vi "fp display engine.vi"(7 "channel data in":sgl[][][](array[numeric]), 10 "Image Refs In":T1[](array[typedef]), 11 "DisplayRefsIn(generic class)":refnum<vi>[](array[refnum])) -> ()   [LabVIEW 2017]
doc: "SciScan 1.2 160622"
uses:
  <vilib>/vision/Image Controls.llb/IMAQ Image.ctl
  Custom Controls/MAIN Image panel tab Control type def.ctl
  Custom Controls/Image Types.ctl
  Custom Controls/scan mode main settings tab.ctl
  Custom Controls/Ch selector.ctl
  GFG/GFGbooleanGet.vi
  GFG/GFGfpRefGet.vi
  <vilib>/vision/NI_Vision_Development_Module.lvlib
  GFG/GFG library.lvlib
panel:
  in  "ROI colors":u32[](array[colorbox])=[6618880, 16716362, 16860, 16776793, 16750848, 16448250, 16716530, 9567230, 16764108, 7340212, 32639, 0, 13816530, 8421376, 8421631, 7171459, 6618880, 16716362, 16860, 16776793, 16750848, 16448250, 16716530, 9567230, 16764108, 7340212, 32639, 0, 13816530, 8421376, 8421631, 7171459, 6618880, 16716362, 16860, 16776793, 16750848, 16448250, 16716530, 9567230, 16764108, 7340212, 32639, 0, 13816530, 8421376, 8421631, 7171459, 6618880, 16716362, 16860, 16776793, 16750848, 16448250, 16716530, 9567230, 16764108, 7340212, 32639, 0, 13816530, 8421376, 8421631, 7171459, 6618880, 16716362, 16860, 16776793, 16750848, 16448250, 16716530, 9567230, 16764108, 7340212, 32639, 0, 13816530, 8421376, 8421631, 7171459, 6618880, 16716362, 16860, 16776793, 16750848, 16448250, 16716530, 9567230, 16764108, 7340212, 32639, 0, 13816530, 8421376, 8421631, 7171459, 6618880, 16716362, 16860, 16776793, 16750848, 16448250, 16716530, 9567230, 16764108, 7340212, 32639, 0, 13816530, 8421376, 8421631, 7171459, 6618880, 16716362, 16860, 16776793, 16750848, 16448250, 16716530, 9567230, 16764108, 7340212, 32639, 0, 13816530, 8421376, 8421631, 7171459, 6618880, 16716362, 16860, 16776793, 16750848, 16448250, 16716530, 9567230, 16764108, 7340212, 32639, 0, 13816530, 8421376, 8421631, 7171459, 6618880, 16716362, 16860, 16776793, 16750848, 16448250, 16716530, 9567230, 16764108, 7340212, 32639, 0, 13816530, 8421376, 8421631, 7171459, 6618880, 16716362, 16860, 16776793, 16750848, 16448250, 16716530, 9567230, 16764108, 7340212, 32639, 0, 13816530, 8421376, 8421631, 7171459, 6618880, 16716362, 16860, 16776793, 16750848, 16448250, 16716530, 9567230, 16764108, 7340212, 32639, 0, 13816530, 8421376, 8421631, 7171459, 6618880, 16716362, 16860, 16776793, 16750848, 16448250, 16716530, 9567230, 16764108, 7340212, 32639, 0, 13816530, 8421376, 8421631, 7171459, 6618880, 16716362, 16860, 16776793, 16750848, 16448250, 16716530, 9567230, 16764108, 7340212, 32639, 0, 13816530, 8421376, 8421631, 7171459, 6618880, 16716362, 16860, 16776793, 16750848, 16448250, 16716530, 9567230, 16764108, 7340212, 32639, 0, 13816530, 8421376, 8421631, 7171459, 6618880, 16716362, 16860, 16776793, 16750848, 16448250, 16716530, 9567230, 16764108, 7340212, 32639, 0, 13816530, 8421376, 8421631, 7171459, 6618880, 16716362, 16860, 16776793, 16750848, 16448250, 16716530, 9567230, 16764108, 7340212, 32639, 0, 13816530, 8421376, 8421631, 7171459, 6618880, 16716362, 16860, 16776793, 16750848, 16448250, 16716530, 9567230, 16764108, 7340212, 32639, 0, 13816530, 8421376, 8421631, 7171459, 6618880, 16716362, 16860, 16776793, 16750848, 16448250, 16716530, 9567230, 16764108, 7340212, 32639, 0, 13816530, 8421376, 8421631, 7171459, 6618880, 16716362, 16860, 16776793, 16750848, 16448250, 16716530, 9567230, 16764108, 7340212, 32639, 0, 13816530, 8421376, 8421631, 7171459, 6618880, 16716362, 16860, 16776793, 16750848, 16448250, 16716530, 9567230, 16764108, 7340212, 32639, 0, 13816530, 8421376, 8421631, 7171459, 6618880, 16716362, 16860, 16776793, 16750848, 16448250, 16716530, 9567230, 16764108, 7340212, 32639, 0, 13816530, 8421376, 8421631, 7171459, 6618880, 16716362, 16860, 16776793, 16750848, 16448250, 16716530, 9567230, 16764108, 7340212, 32639, 0, 13816530, 8421376, 8421631, 7171459, 6618880, 16716362, 16860, 16776793, 16750848, 16448250, 16716530, 9567230, 16764108, 7340212, 32639, 0, 13816530, 8421376, 8421631, 7171459, 6618880, 16716362, 16860, 16776793, 16750848, 16448250, 16716530, 9567230, 16764108, 7340212, 32639, 0, 13816530, 8421376, 8421631, 7171459]
  out "error out":errorcluster
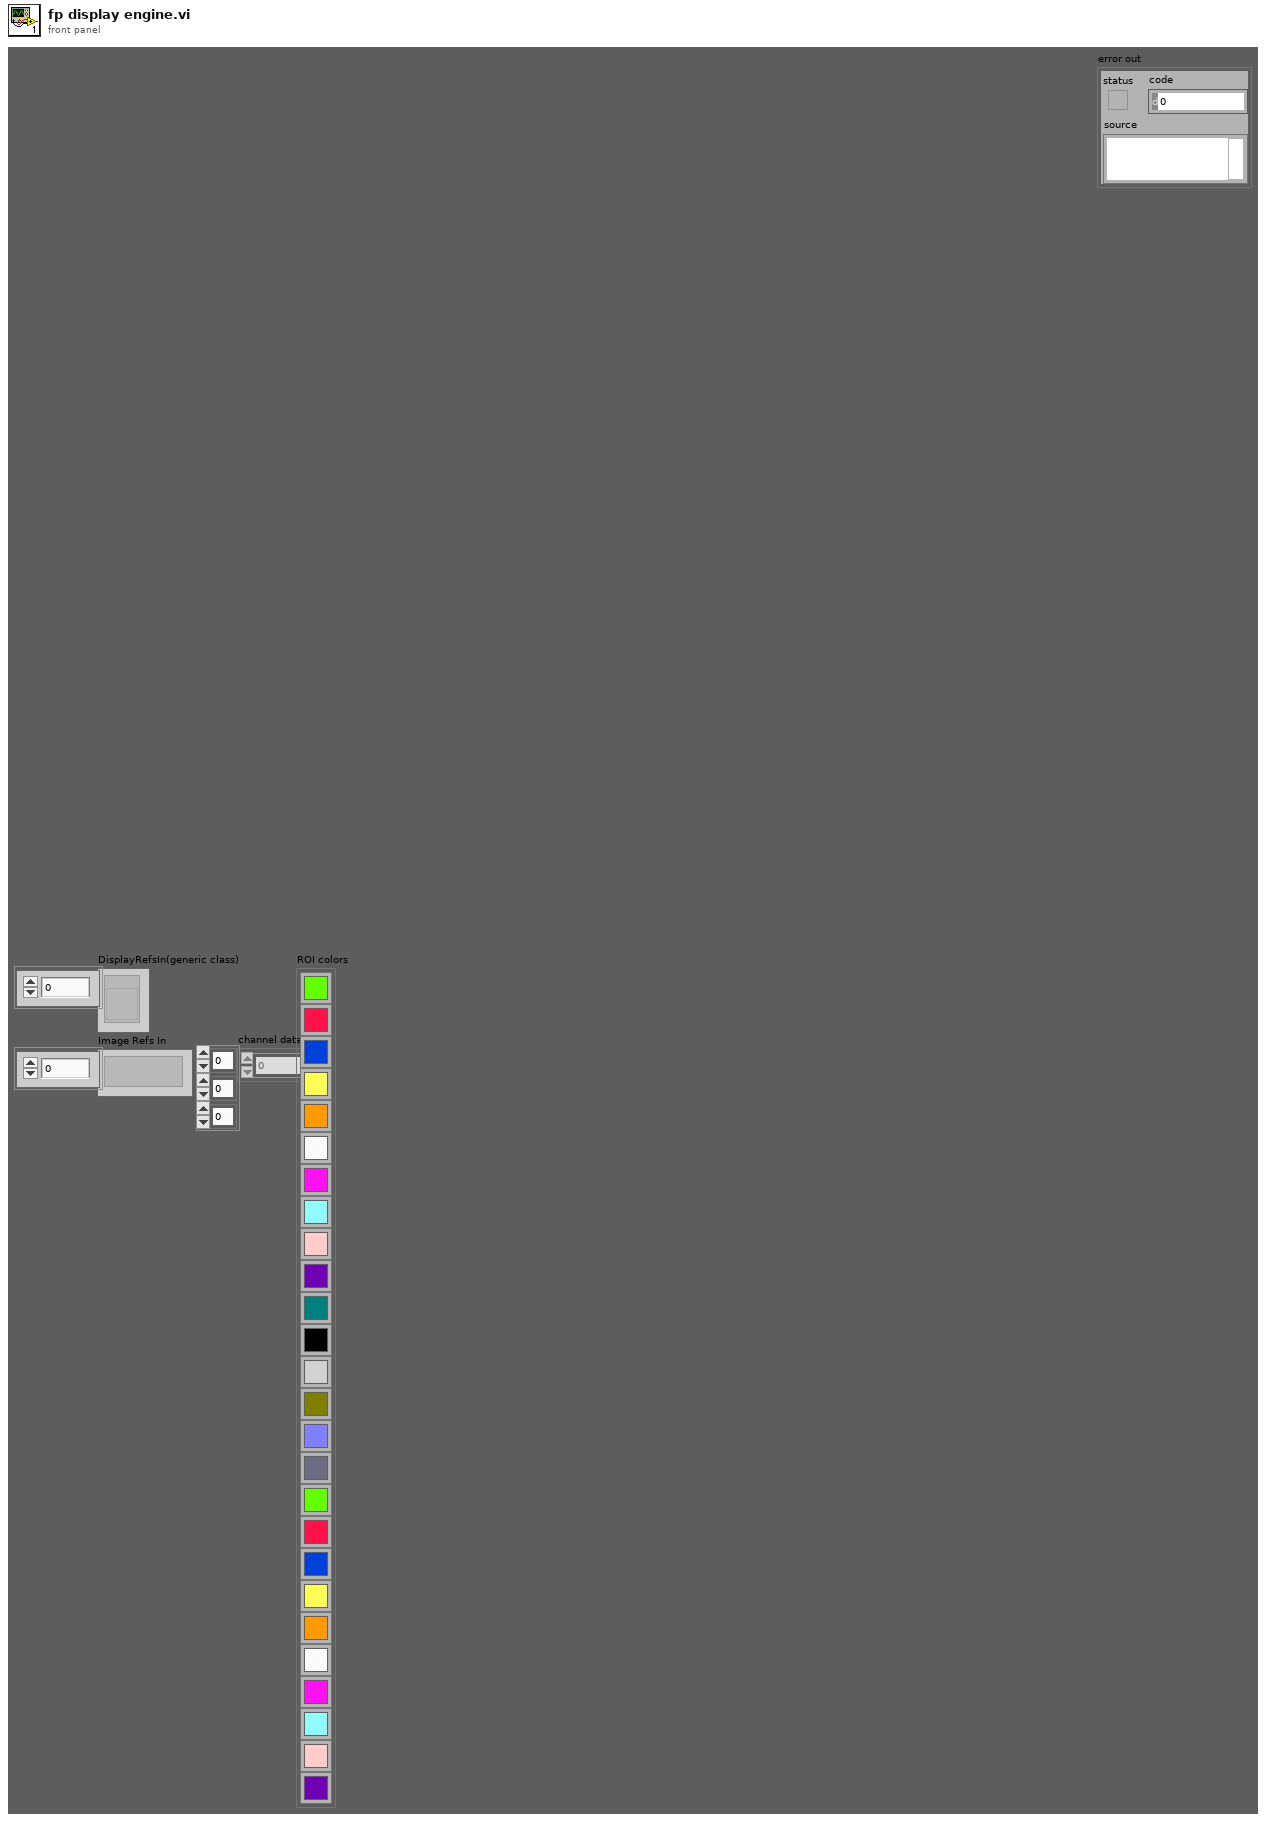
[diagram p1: front panel]
types:
  T1 = typedef "IMAQ Image.ctl" = refnum<image>
  T2 = typedef "MAIN Image panel tab Control type def.ctl" = enum32{"Channel 1", "Channel 2", "Channel 3", "Channel 4", "all channels", "RGB overlay", "ROI", "arbitrary line scan"}
  T3 = enum32{"Channel 1", "Channel 2", "Channel 3", "Channel 4", "Channel 5", "all channels", "RGB overlay", "ROI", "arbitrary line scan"}
  T4 = typedef "Image Types.ctl" = enum16{"Frame Scan", "Line Scan", "RGB Overlay", "ROI", "All Channels Frame"}
  T5 = typedef "scan mode main settings tab.ctl" = enum32{"2D frame", "2D line scan", "general settings", "Z Stack", "piezo"}
  T6 = typedef "Ch selector.ctl" = enum16{"none", "Ch 1", "Ch 2", "Ch 3", "Ch 4"}
  T7 = typedef "Image Type" = u32
  T8 = cluster{"Global Rectangle":i32[], "Contours":cluster{"Contour Type":u32, "ROI Type":u32, "Points":i32[]}[]}
  T9 = typedef "ROI Descriptor" = cluster{"Global Rectangle":i32[], "Contours":cluster{"ID":enum32{"External", "Internal"}, "Type":u32, "Coordinates":i32[]}[]}
  T10 = cluster{"WaveformChartRef":refnum<vi>, "DigitalRef":refnum<vi>, "ArrayRef":refnum<vi>, "TabControlRef":refnum<vi>, "EnumRef":refnum<vi>, "RingRef":refnum<vi>, "BooleanRef":refnum<vi>, "KnobRef":refnum<vi>, "SlideRef":refnum<vi>, "PathRef":refnum<vi>, "StringRef":refnum<vi>, "ComboBox":refnum<vi>, "WaveformGraphRef":refnum<vi>}
  T11 = cluster{"Mean Value":sgl, "Standard Variation":sgl, "Minimal Value":sgl, "Maximal Value":sgl, "Area (calibrated)":sgl, "Area (pixels)":i32, "%":sgl}[]
  T12 = cluster{"Mean Value":sgl, "Standard Variation":sgl, "Minimal Value":sgl, "Maximal Value":sgl, "Area (calibrated)":sgl, "Area (pixels)":i32, "%":sgl}
  T13 = cluster{"Contour Type":u32, "ROI Type":u32, "Points":i32[]}[]
  T14 = cluster{"Starting Value":sgl, "Incremental Value":sgl, "Histogram":u32[]}
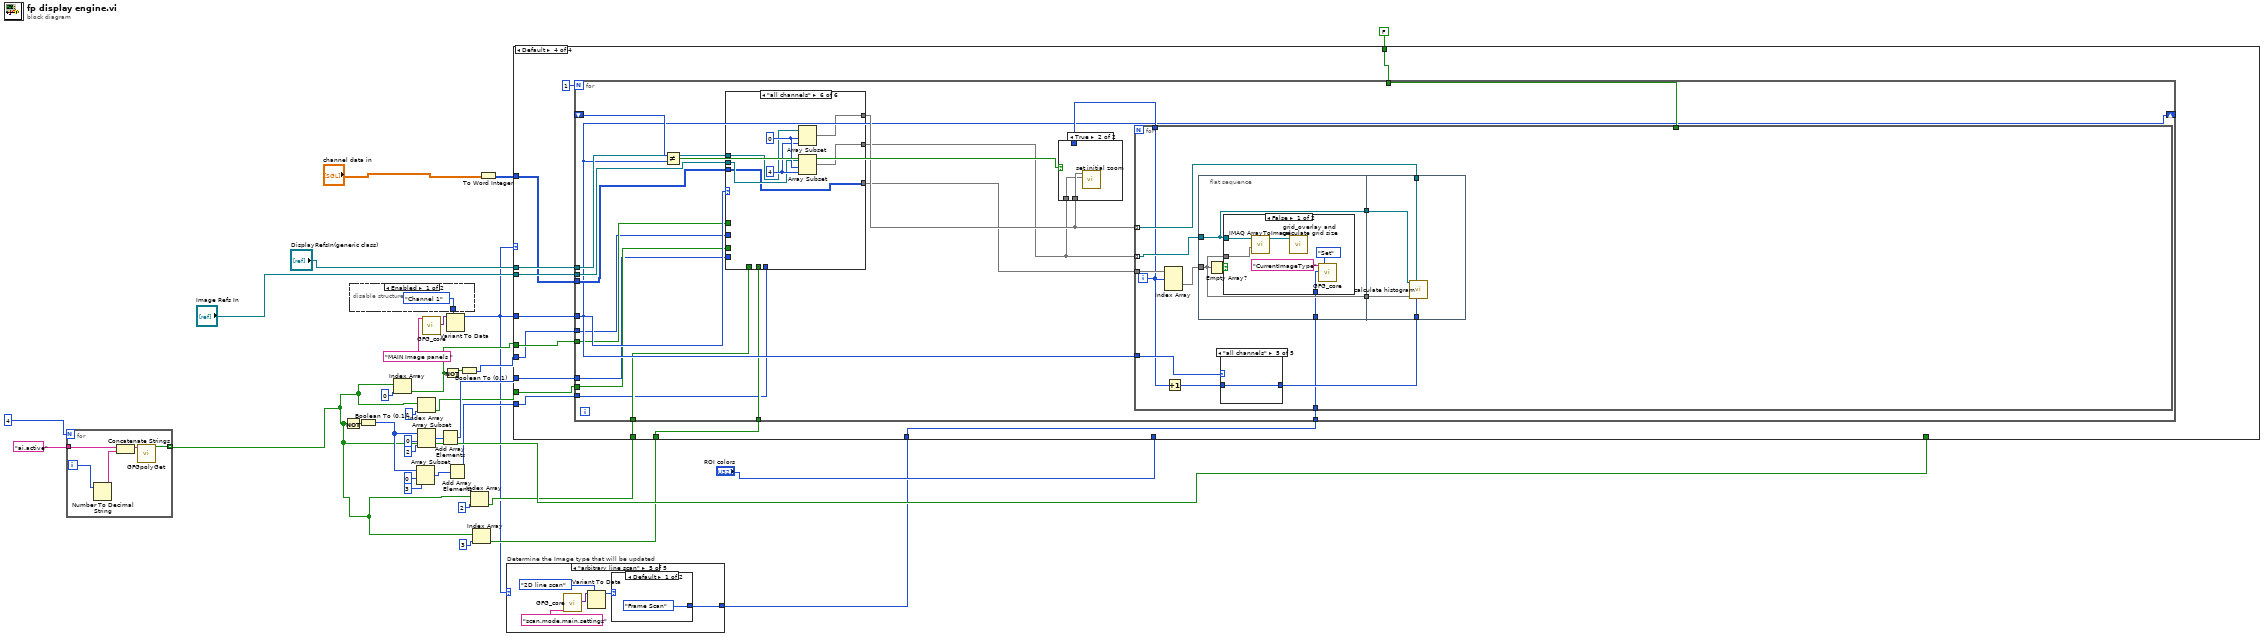
[diagram p0: block diagram]
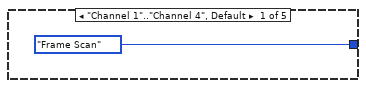
[diagram p2: hidden frame]
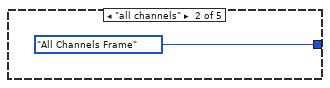
[diagram p3: hidden frame]
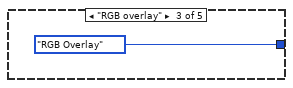
[diagram p4: hidden frame]
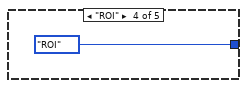
[diagram p5: hidden frame]
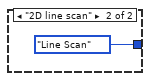
[diagram p6: hidden frame]
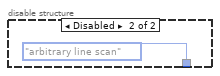
[diagram p7: hidden frame]
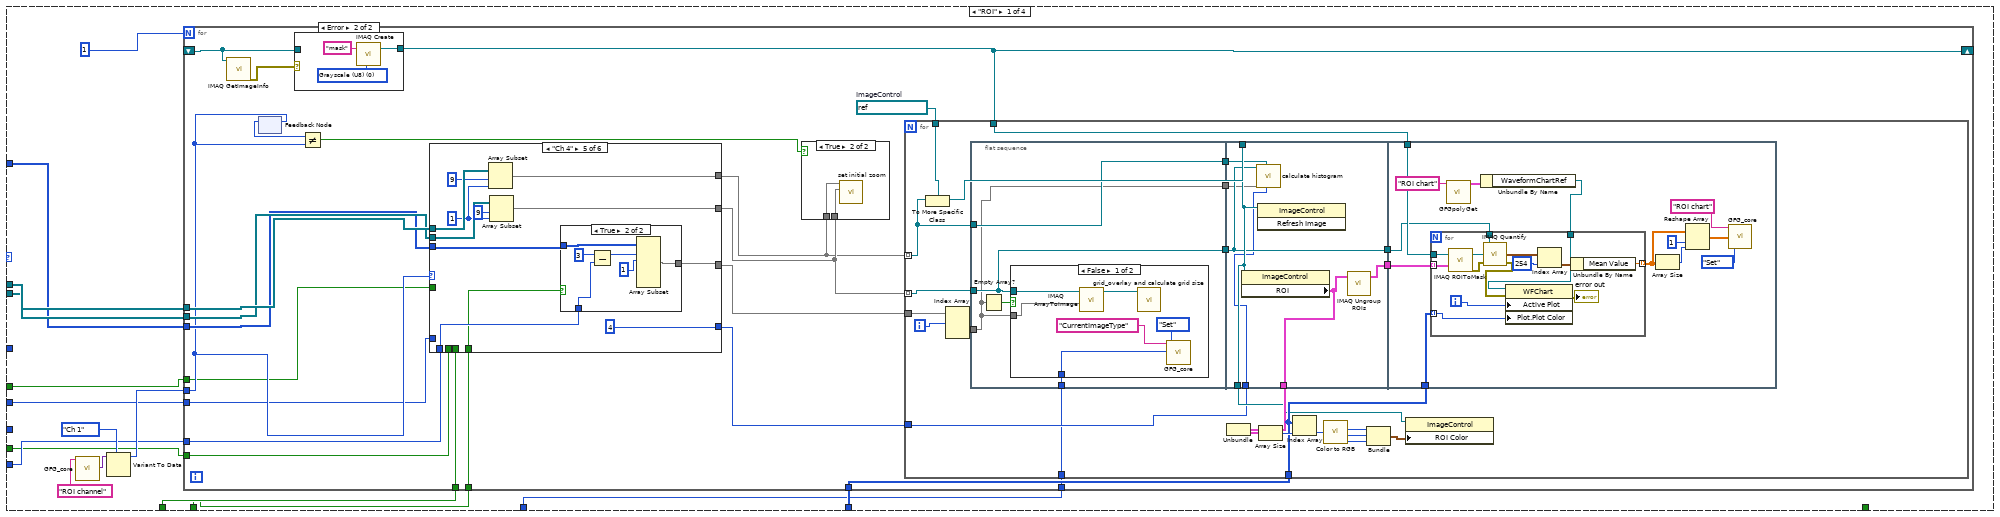
[diagram p8: hidden frame]
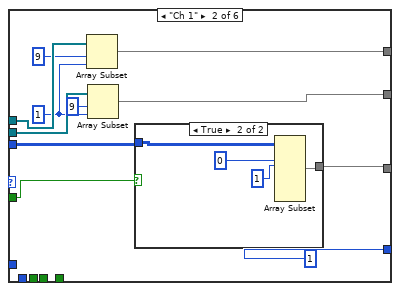
[diagram p10: hidden frame]
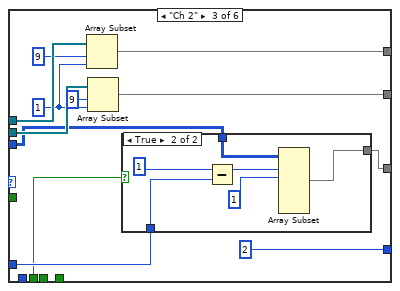
[diagram p12: hidden frame]
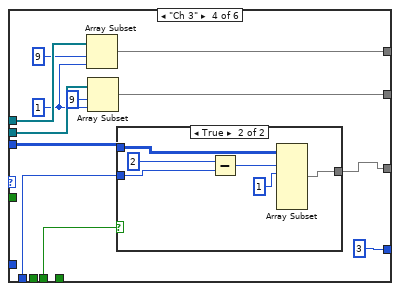
[diagram p14: hidden frame]
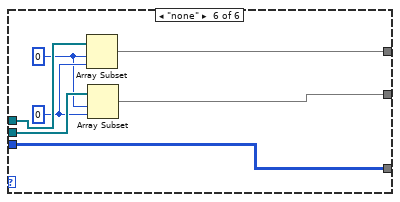
[diagram p17: hidden frame]
diagram:
  n1 = for {
    N: 4 -> [_]
    tunnel: "ai.active" ("Variable Name in") -> [w39]
    tunnel: [w38] -> w10 mode=indexing
    i -> [w35]
    n2 = Number To Decimal String(number=w35) -> (decimal integer string=w36:string)  [unwired: 1 in]
    n3 = Concatenate Strings(w39, w36) -> (w37:string)
    n4 = call-poly "GFGpolyGet.vi"("Variable Name in"=w37) -> ("Boolean Value OUT"=w38:bool)  [unwired: 9 in, 1 out]
  }
  n5 = Not(x=w10) -> (.not. x?=w17:bool[])
  n6 = disable-structure shown="Enabled" {
    disable-tunnel: [MAIN_Image_panel_tab_Control_type_def."Channel 1" ("MAIN Image panels") T3."arbitrary line scan" ("MAIN Image panels")] -> w32
    frame Enabled {
    }
    frame Disabled {
    }
  }
  n7 = Boolean To (0,1)(Boolean=w17) -> (0, 1=w16:i16[])
  n8 = Index Array(array=w10, index=0) -> (element=w9:bool)
  n9 = Array Subset(array=w16, index=0, length=3) -> (w19:i16[])
  n10 = Array Subset(array=w16, index=0, length=2) -> (w18:i16[])
  n11 = Index Array(array=w10, index=1) -> (element=w6:bool)
  n12 = call "GFG_core.vi"("Variable Name in"="MAIN Image panels ") -> ("Variant Out"=w34:variant)  [unwired: 12 in, 6 out]
  n13 = Add Array Elements(numeric array=w18) -> (sum=w7:i16)
  n14 = Not(x=w9) -> (.not. x?=w20:bool)
  n15 = Variant To Data(type=w32, Variant=w34) -> (data=w2:T2)  [unwired: 1 in, 1 out]
  n16 = Add Array Elements(numeric array=w19) -> (sum=w5:i16)
  n17 = Boolean To (0,1)(Boolean=w20) -> (0, 1=w8:i16)
  n18 = Index Array(array=w10, index=2) -> (element=w4:bool)
  n19 = Index Array(array=w10, index=3) -> (element=w3:bool)
  n20 = To Word Integer(number="channel data in") -> (16bit integer=w28:i16[][][])
  n21 = case "Determine the Image type that will be updated" shown="\"arbitrary line scan\"" w2 {
    tunnel: [Image_Types."Frame Scan" ("Image Types") Image_Types."All Channels Frame" ("Image Types") Image_Types."RGB Overlay" ("Image Types") Image_Types."ROI" ("Image Types") w46] -> w1
    frame "Channel 1".."Channel 4", Default {
    }
    frame "all channels" {
    }
    frame "RGB overlay" {
    }
    frame "ROI" {
    }
    frame "arbitrary line scan" {
      n22 = call "GFG_core.vi"("Variable Name in"="scan.mode.main.settings") -> ("Variant Out"=w49:variant)  [unwired: 12 in, 6 out]
      n23 = Variant To Data(type=scan_mode_main_settings_tab."2D line scan" ("scan mode main settings"), Variant=w49) -> (data=w47:T5)  [unwired: 1 in, 1 out]
      n24 = case shown="Default" w47 {
        tunnel: [Image_Types."Frame Scan" ("Image Types") Image_Types."Line Scan" ("Image Types")] -> w46
        frame Default {
        }
        frame "2D line scan" {
        }
      }
    }
  }
  n25 = case shown="Default" w2 {
    tunnel: w2 -> [_ _ _ w476]
    tunnel: "DisplayRefsIn(generic class)" -> [w67 w253 w392 w479]
    tunnel: "Image Refs In" -> [w66 w252 w383 w478]
    tunnel: w28 -> [w65 w251 w391 w477]
    tunnel: FALSE -> [_ _ w390 w474]
    tunnel: "ROI colors" -> [w61 _ _ _]
    tunnel: w10 -> [_ _ w377 _]
    tunnel: w9 -> [w59 _ _ w468]
    tunnel: w8 -> [w58 w246 _ w467]
    tunnel: w7 -> [_ w245 _ w469]
    tunnel: w6 -> [w56 _ _ w470]
    tunnel: w5 -> [w57 w244 _ w471]
    tunnel: w4 -> [w55 _ _ w472]
    tunnel: w3 -> [w54 _ _ w473]
    tunnel: w1 -> [w53 w243 w376 w466]
    frame "ROI" {
      n26 = call "GFG_core.vi"("Variable Name in"="ROI channel") -> ("Variant Out"=w63:variant)  [unwired: 12 in, 6 out]
      n27 = Variant To Data(type=Ch_selector."Ch 1" ("ROI channel"), Variant=w63) -> (data=w62:T6)  [unwired: 1 in, 1 out]
      n28 = for {
        N: 1 -> [_]
        tunnel: w67 -> [w83]
        tunnel: w66 -> [w82]
        tunnel: w65 -> [w81]
        tunnel: w62 -> [w80]
        shift-right: [w87] -> _
        shift-left: _ -> [w86]
        tunnel: w61 -> [w84]
        tunnel: w59 -> [w75]
        tunnel: w58 -> [w74]
        tunnel: w57 -> [w73]
        tunnel: w56 -> [w72]
        tunnel: w55 -> [w71]
        tunnel: w54 -> [w70]
        tunnel: w53 -> [w69]
        w90 = refnum<vi> refnum  # ImageControl
        n29 = call "IMAQ GetImageInfo"("Image"=w86) -> ("error out"=w85:errorcluster)  [unwired: 3 in, 7 out]
        n30 = feedback-in #1(w80) -> ()
        n31 = feedback #1() -> (w89:T6)  [unwired: 1 in]
        n32 = case shown="Error" w85 {
          tunnel: [w167 w168] -> w87
          tunnel: w86 -> [w167 _]
          frame No Error {
          }
          frame Error {
            w169 = T7 0 items=["Grayscale (U8)", "Grayscale (I16)", "Grayscale (SGL)", "Complex (CSG)", "RGB (U32)", "HSL (U32)", "RGB (U64)"] ("Image Type")
            n33 = call "IMAQ Create"("Image Name"="mask", "Image Type"=w169) -> ("New Image"=w168:T1)  [unwired: 3 in, 1 out]
          }
        }
        n34 = Not Equal?(x=w89, y=w80) -> (x != y?=w88:bool)
        n35 = case shown="\"Ch 4\"" w80 {
          tunnel: w83 -> [_ w100 w116 w134 w152 w165]
          tunnel: w82 -> [_ w101 w117 w135 w153 w166]
          tunnel: [_ w97 w113 w131 w149 w162] -> w78
          tunnel: [_ w96 w112 w130 w148 w161] -> w77
          tunnel: w81 -> [_ w93 w109 w126 w144 w160]
          tunnel: [_ w91 w108 w127 w145 w160] -> w79
          tunnel: [_ 1 ("length") 2 ("length") 3 ("length") 4 ("length") _] -> w76
          tunnel: w75 -> [_ w92 _ _ _ _]
          tunnel: w74 -> [_ _ w107 _ _ _]
          tunnel: w72 -> [_ _ w106 _ _ _]
          tunnel: w73 -> [_ _ _ w125 w143 _]
          tunnel: w71 -> [_ _ _ w124 _ _]
          tunnel: w70 -> [_ _ _ _ w142 _]
          frame Default {
          }
          frame "Ch 1" {
            w99 = 1 ("length")
            n36 = Array Subset(array=w100, index=9, length=w99) -> (w96:refnum<vi>[])
            n37 = Array Subset(array=w101, index=9, length=w99) -> (w97:T1[])
            n38 = case shown="True" w92 {
              tunnel: w93 -> [_ w105]
              tunnel: [_ w103] -> w91
              frame False {
              }
              frame True {
                n39 = Array Subset(array=w105, index (dim 0)=0 ("index"), length (dim 0)=1 ("length")) -> (w103:i16[][][])  [unwired: 4 in]
              }
            }
          }
          frame "Ch 2" {
            w115 = 1 ("length")
            n40 = Array Subset(array=w116, index=9, length=w115) -> (w112:refnum<vi>[])
            n41 = Array Subset(array=w117, index=9, length=w115) -> (w113:T1[])
            n42 = case shown="True" w106 {
              tunnel: w109 -> [_ w121]
              tunnel: [_ w120] -> w108
              tunnel: w107 -> [_ w118]
              frame False {
              }
              frame True {
                n43 = Subtract(x=1 ("index"), y=w118) -> (x-y=w119:i32)
                n44 = Array Subset(array=w121, index (dim 0)=w119, length (dim 0)=1 ("length")) -> (w120:i16[][][])  [unwired: 4 in]
              }
            }
          }
          frame "Ch 3" {
            w132 = 1 ("index")
            n45 = Array Subset(array=w134, index=9, length=w132) -> (w130:refnum<vi>[])
            n46 = Array Subset(array=w135, index=9, length=w132) -> (w131:T1[])
            n47 = case shown="True" w124 {
              tunnel: w126 -> [_ w140]
              tunnel: [_ w139] -> w127
              tunnel: w125 -> [_ w137]
              frame False {
              }
              frame True {
                n48 = Subtract(x=2 ("index"), y=w137) -> (x-y=w138:i32)
                n49 = Array Subset(array=w140, index (dim 0)=w138, length (dim 0)=1 ("length")) -> (w139:i16[][][])  [unwired: 4 in]
              }
            }
          }
          frame "Ch 4" {
            w151 = 1 ("index")
            n50 = Array Subset(array=w152, index=9, length=w151) -> (w148:refnum<vi>[])
            n51 = Array Subset(array=w153, index=9, length=w151) -> (w149:T1[])
            n52 = case shown="True" w142 {
              tunnel: w144 -> [_ w158]
              tunnel: [_ w157] -> w145
              tunnel: w143 -> [_ w154]
              frame False {
              }
              frame True {
                n53 = Subtract(x=3 ("index"), y=w154) -> (x-y=w156:i32)
                n54 = Array Subset(array=w158, index (dim 0)=w156, length (dim 0)=1 ("length")) -> (w157:i16[][][])  [unwired: 4 in]
              }
            }
          }
          frame "none" {
            w163 = 0 ("index")
            w164 = 0 ("length")
            n55 = Array Subset(array=w165, index=w163, length=w164) -> (w161:refnum<vi>[])
            n56 = Array Subset(array=w166, index=w163, length=w164) -> (w162:T1[])
          }
        }
        n57 = case shown="True" w88 {
          tunnel: w77 -> [_ w172]
          tunnel: w78 -> [_ w171]
          frame False {
          }
          frame True {
            n58 = call "set initial zoom.vi"("Image Refs In"=w171, "DisplayRefsIn(generic class)"=w172) -> ()  [unwired: 10 in]
          }
        }
        n59 = for {
          tunnel: w77 -> [w176] mode=indexing
          tunnel: w78 -> [w195] mode=indexing
          tunnel: w79 -> [w197]
          tunnel: w90 -> [w194]
          tunnel: w87 -> [w179]
          tunnel: w84 -> [w182]
          tunnel: w76 -> [w174]
          tunnel: w69 -> [w173]
          i -> [w192]
          n60 = To More Specific Class(target class=w194, reference=w176) -> (specific class reference=w193:refnum<vi>)  [unwired: 1 in, 1 out]
          n61 = Index Array(array=w197, index (dim 0)=w192) -> (element=w196:i16[][])  [unwired: 2 in]
          n62 = flat-sequence {
            tunnel: w196 -> [w199]
            tunnel: w195 -> [w201]
            tunnel: [w201] -> w180
            tunnel: [w200] -> w177
            tunnel: w176 -> [w200]
            tunnel: [w199] -> w175
            tunnel: w173 -> [w198]
            tunnel: w193 -> [w213]
            tunnel: [w215] -> w185
            tunnel: [w214] -> w183
            tunnel: [w211] -> w181
            tunnel: w180 -> [w211]
            tunnel: [w213] -> w178
            tunnel: w177 -> [w212]
            tunnel: w175 -> [w210]
            tunnel: w174 -> [w209]
            tunnel: w183 -> [w225]
            tunnel: w182 -> [w224]
            tunnel: w181 -> [w216]
            tunnel: w179 -> [w217]
            frame #0 {
              n63 = Empty Array?(array=w199) -> (empty?=w202:bool)
              n64 = case shown="False" w202 {
                tunnel: w201 -> [w208 _]
                tunnel: w199 -> [w207 _]
                tunnel: w198 -> [w203 _]
                frame False {
                  n65 = call "IMAQ ArrayToImage"("Image Pixels (I16)"=w207, "Image"=w208) -> ("Image Out"=w206:T1)  [unwired: 8 in, 1 out]
                  n66 = call "grid_overlay and calculate grid size.vi"("Image In"=w206) -> ()  [unwired: 10 in, 1 out]
                  n67 = call "GFG_core.vi"("Variable Name in"="CurrentImageType", "Variant in"=w203, "Action"=enum16{"Init", "Set", "Get", "Clear"}."Set") -> ()  [unwired: 10 in, 7 out]
                }
                frame True {
                }
              }
            }
            frame #1 {
              n68 = property class="ImageControl"(reference=w213) -> ("ROI"=w215:T8)  [unwired: 1 in, 2 out]
              n69 = call "calculate histogram.vi"("channel no."=w209, "Image Ctrl Ref (as generic class)"=w212, "Image Array"=w210, "Image"=w211) -> ()  [unwired: 8 in]
              n70 = invoke class="ImageControl" method="Refresh Image"(reference=w213) -> ()  [unwired: 2 in, 3 out]
              n71 = call "IMAQ Ungroup ROIs"("ROI Descriptor"=w215) -> ("ROI Descriptors out"=w214:T9[])  [unwired: 3 in, 1 out]
            }
            frame #2 {
              n72 = call-poly "GFGpolyGet.vi"("Variable Name in"="ROI chart") -> ("output cluster"=w219:T10)  [unwired: 9 in, 1 out]
              n73 = Unbundle By Name(w219) -> ("WaveformChartRef"=w218:refnum<vi>)
              n74 = for {
                tunnel: w216 -> [w242]
                tunnel: w225 -> [w236] mode=indexing
                tunnel: [w238] -> w228 mode=indexing
                tunnel: w217 -> [w235]
                tunnel: w224 -> [w232] mode=indexing
                tunnel: w218 -> [w231]
                i -> [w233]
                n75 = call "IMAQ ROIToMask"("ROI Descriptor"=w236, "Image"=w235) -> ("error out"=w230:errorcluster, "Image Out"=w237:T1)  [unwired: 4 in, 1 out]
                n76 = call "IMAQ Quantify"("error in (no error)"=w230, "Image Mask"=w237, "Image"=w242) -> ("error out"=w229:errorcluster, "Region Reports"=w241:T11)  [unwired: 1 out]
                n77 = property on="Property Node" class="WFChart"(reference=w231, error in=w229, "Active Plot"=w233, "Plot.Plot Color"=w232) -> (error out=→"error out":errorcluster)  [unwired: 1 out]
                n78 = Index Array(array=w241, index=254) -> (element=w239:T12)
                n79 = Unbundle By Name(w239) -> ("Mean Value"=w238:sgl)
              }
              n80 = Array Size(array=w228) -> (size(s)=w227:i32)
              n81 = Reshape Array(w228, 1 ("dimension size"), w227) -> (w222:sgl[][])
              n82 = call "GFG_core.vi"("Variable Name in"="ROI chart", "Variant in"=w222, "Action"=enum16{"Init", "Set", "Get"}."Set") -> ()  [unwired: 10 in, 7 out]
            }
          }
          n83 = Unbundle(w185) -> ("Contours"=w190:T13)  [unwired: 1 out]
          n84 = Array Size(array=w190) -> (size(s)=w191:i32)
          n85 = Index Array(array=w182, index=w191) -> (element=w186:u32)
          n86 = call <vilib>:"Color to RGB.vi"("Color"=w186) -> ("R"=w187:u8, "G"=w188:u8, "B"=w189:u8)  [unwired: 1 out]
          n87 = Bundle("R"=w187, "G"=w188, "B"=w189) -> (w184:cluster{"R":u8, "G":u8, "B":u8})  [unwired: 1 in]
          n88 = property class="ImageControl"(reference=w178, "ROI Color"=w184) -> ()  [unwired: 1 in, 2 out]
        }
      }
    }
    frame "arbitrary line scan" {
      n89 = call "GFG_core.vi"("Variable Name in"="channel arb line scan") -> ("Variant Out"=w249:variant)  [unwired: 12 in, 6 out]
      n90 = Variant To Data(type=Ch_selector."Ch 1" ("ROI channel"), Variant=w249) -> (data=w248:T6)  [unwired: 1 in, 1 out]
      n91 = for {
        N: 1 -> [_]
        tunnel: w253 -> [w268]
        tunnel: w252 -> [w267]
        tunnel: w251 -> [w266]
        tunnel: w248 -> [w263]
        tunnel: w246 -> [w258]
        tunnel: w245 -> [w257]
        tunnel: w244 -> [w256]
        tunnel: w243 -> [w255]
        w265 = refnum<vi> refnum  # ImageControl
        n92 = case shown="\"none\"" w263 {
          tunnel: w268 -> [_ w282 w296 w310 w324 w331]
          tunnel: w267 -> [_ w283 w297 w311 w325 w332]
          tunnel: [_ w279 w293 w307 w321 w328] -> w259
          tunnel: [_ w278 w292 w306 w320 w327] -> w262
          tunnel: w266 -> [_ w277 w289 w303 w317 w326]
          tunnel: [_ w274 w288 w302 w316 w326] -> w269
          tunnel: [_ 1 ("length") 2 ("length") 3 ("length") 4 ("length") _] -> w260
          tunnel: w258 -> [_ _ w284 _ _ _]
          tunnel: w257 -> [_ _ _ w298 _ _]
          tunnel: w256 -> [_ _ _ _ w312 _]
          frame Default {
          }
          frame "Ch 1" {
            w281 = 1 ("length")
            n93 = Array Subset(array=w282, index=10, length=w281) -> (w278:refnum<vi>[])
            n94 = Array Subset(array=w283, index=10, length=w281) -> (w279:T1[])
            n95 = Array Subset(array=w277, index (dim 0)=0 ("index"), length (dim 0)=1 ("length")) -> (w274:i16[][][])  [unwired: 4 in]
          }
          frame "Ch 2" {
            w295 = 1 ("length")
            n96 = Subtract(x=1 ("index"), y=w284) -> (x-y=w285:i32)
            n97 = Array Subset(array=w296, index=10, length=w295) -> (w292:refnum<vi>[])
            n98 = Array Subset(array=w297, index=10, length=w295) -> (w293:T1[])
            n99 = Array Subset(array=w289, index (dim 0)=w285, length (dim 0)=1 ("length")) -> (w288:i16[][][])  [unwired: 4 in]
          }
          frame "Ch 3" {
            w308 = 1 ("index")
            n100 = Subtract(x=2 ("index"), y=w298) -> (x-y=w299:i32)
            n101 = Array Subset(array=w310, index=10, length=w308) -> (w306:refnum<vi>[])
            n102 = Array Subset(array=w311, index=10, length=w308) -> (w307:T1[])
            n103 = Array Subset(array=w303, index (dim 0)=w299, length (dim 0)=1 ("length")) -> (w302:i16[][][])  [unwired: 4 in]
          }
          frame "Ch 4" {
            w323 = 1 ("index")
            n104 = Subtract(x=3 ("index"), y=w312) -> (x-y=w313:i32)
            n105 = Array Subset(array=w324, index=10, length=w323) -> (w320:refnum<vi>[])
            n106 = Array Subset(array=w325, index=10, length=w323) -> (w321:T1[])
            n107 = Array Subset(array=w317, index (dim 0)=w313, length (dim 0)=1 ("length")) -> (w316:i16[][][])  [unwired: 4 in]
          }
          frame "none" {
            w329 = 0 ("index")
            w330 = 0 ("length")
            n108 = Array Subset(array=w331, index=w329, length=w330) -> (w327:refnum<vi>[])
            n109 = Array Subset(array=w332, index=w329, length=w330) -> (w328:T1[])
          }
        }
        n110 = feedback-in #2(w263) -> ()
        n111 = feedback #2() -> (w264:T6)  [unwired: 1 in]
        n112 = Not Equal?(x=w264, y=w263) -> (x != y?=w261:bool)
        n113 = case shown="True" w261 {
          tunnel: w262 -> [_ w271]
          tunnel: w259 -> [_ w270]
          frame False {
          }
          frame True {
            n114 = call "set initial zoom.vi"("Image Refs In"=w270, "DisplayRefsIn(generic class)"=w271) -> ()  [unwired: 10 in]
          }
        }
        n115 = for {
          tunnel: w262 -> [w337] mode=indexing
          tunnel: w259 -> [w344] mode=indexing
          tunnel: w269 -> [w346]
          tunnel: w265 -> [w343]
          tunnel: w260 -> [w335]
          tunnel: w255 -> [w333]
          i -> [w341]
          n116 = To More Specific Class(target class=w343, reference=w337) -> (specific class reference=w342:refnum<vi>)  [unwired: 1 in, 1 out]
          n117 = Index Array(array=w346, index (dim 0)=w341) -> (element=w345:i16[][])  [unwired: 2 in]
          n118 = flat-sequence {
            tunnel: w345 -> [w348]
            tunnel: w344 -> [w350]
            tunnel: [w350] -> w339
            tunnel: [w349] -> w338
            tunnel: w337 -> [w349]
            tunnel: [w348] -> w336
            tunnel: w333 -> [w347]
            tunnel: w342 -> [w358]
            tunnel: [w363] -> w340
            tunnel: w339 -> [w361]
            tunnel: [w358] -> _
            tunnel: w338 -> [w362]
            tunnel: w336 -> [w360]
            tunnel: w335 -> [w359]
            tunnel: [w358] -> w334
            tunnel: w340 -> [w369]
            tunnel: w334 -> [w368]
            frame #0 {
              n119 = Empty Array?(array=w348) -> (empty?=w351:bool)
              n120 = case shown="False" w351 {
                tunnel: w350 -> [w356 _]
                tunnel: w348 -> [w355 _]
                tunnel: w347 -> [w352 _]
                frame False {
                  n121 = call "IMAQ ArrayToImage"("Image Pixels (I16)"=w355, "Image"=w356) -> ()  [unwired: 8 in, 2 out]
                  n122 = call "GFG_core.vi"("Variable Name in"="CurrentImageType", "Variant in"=w352, "Action"=enum16{"Init", "Set", "Get", "Clear"}."Set") -> ()  [unwired: 10 in, 7 out]
                }
                frame True {
                }
              }
            }
            frame #1 {
              n123 = call "calculate histogram.vi"("channel no."=w359, "Image Ctrl Ref (as generic class)"=w362, "Image Array"=w360, "Image"=w361) -> ()  [unwired: 8 in]
              n124 = property class="ImageControl"(reference=w358) -> ("ROI"=w357:T8)  [unwired: 1 in, 2 out]
              n125 = call "IMAQ Ungroup ROIs"("ROI Descriptor"=w357) -> ("ROI Descriptors out"=w363:T9[])  [unwired: 3 in, 1 out]
            }
            frame #2 {
              n126 = for {
                tunnel: w369 -> [w375] mode=indexing
                tunnel: [w375] -> w364
                tunnel: [w374] -> w367
                i -> [w374]
              }
              n127 = Greater?(x=w367, y=1) -> (0:w365:bool)
              n128 = case shown="True" w365 {
                tunnel: w364 -> [_ w373]
                tunnel: w368 -> [_ w370]
                frame False {
                }
                frame True {
                  n129 = Build Array(w373) -> (w372:T9[])
                  n130 = call "IMAQ Group ROIs"("ROI Descriptors"=w372) -> ("ROI Descriptor out"=w371:T9)  [unwired: 3 in, 1 out]
                  n131 = property class="ImageControl"(reference=w370, "ROI"=w371) -> ()  [unwired: 1 in, 2 out]
                }
              }
            }
          }
        }
      }
    }
    frame "RGB overlay" {
      w378 = refnum<vi> refnum  # ImageControl
      n132 = Array Subset(array=w383, index=8, length=1) -> (w382:T1[])
      n133 = Array Subset(array=w392, index=8, length=1) -> (w379:refnum<vi>[])
      n134 = Array Subset(array=w383, index=0, length=4) -> (w380:T1[])
      n135 = disable-structure shown="Disabled" {
        disable-tunnel: w380 -> [w394 _]
        disable-tunnel: w379 -> [w393 _]
        frame Disabled {
          n136 = call "set initial zoom.vi"("Image Refs In"=w394, "DisplayRefsIn(generic class)"=w393) -> ()  [unwired: 10 in]
        }
        frame Enabled {
        }
      }
      n137 = for {
        tunnel: w380 -> [w418] mode=indexing
        tunnel: w391 -> [w420]
        tunnel: w390 -> [w411]
        tunnel: [w407] -> w381 mode=indexing
        tunnel: w376 -> [w406]
        i -> [w415]
        n138 = Increment(x=w415) -> (x+1=w413:i32)
        n139 = Index Array(array=w420, index (dim 0)=w415) -> (element=w419:i16[][])  [unwired: 2 in]
        n140 = flat-sequence {
          tunnel: w419 -> [w422]
          tunnel: w418 -> [w423]
          tunnel: [w423] -> w416
          tunnel: [w422] -> w414
          tunnel: w406 -> [w421]
          tunnel: [w435] -> w417
          tunnel: w416 -> [w435]
          tunnel: w414 -> [w430]
          tunnel: [w433] -> w412
          tunnel: [w430] -> w410
          tunnel: w417 -> [w454]
          tunnel: w413 -> [w453]
          tunnel: w412 -> [w441]
          tunnel: w411 -> [w436]
          tunnel: [w438] -> w408
          tunnel: [w437] -> w409
          frame #0 {
            n141 = Empty Array?(array=w422) -> (empty?=w424:bool)
            n142 = case shown="False" w424 {
              tunnel: w423 -> [w429 _]
              tunnel: w422 -> [w428 _]
              tunnel: w421 -> [w425 _]
              frame False {
                n143 = call "IMAQ ArrayToImage"("Image Pixels (I16)"=w428, "Image"=w429) -> ()  [unwired: 8 in, 2 out]
                n144 = call "GFG_core.vi"("Variable Name in"="CurrentImageType", "Variant in"=w425, "Action"=enum16{"Init", "Set", "Get", "Clear"}."Set") -> ()  [unwired: 10 in, 7 out]
              }
              frame True {
              }
            }
          }
          frame #1 {
            n145 = Array Max & Min(array=w430) -> (max value=w434:i16, min value=w432:i16)  [unwired: 2 out]
            n146 = Decrement(x=w434) -> (x-1=w431:i16)
            n147 = Bundle(w432, w431) -> (w433:cluster{i16, i16})  [unwired: 1 in]
          }
          frame #2 {
            n148 = Number To Decimal String(number=w453) -> (decimal integer string=w448:string)  [unwired: 1 in]
            n149 = Concatenate Strings("Histogram " ("string"), w448) -> (w456:string)
            n150 = Concatenate Strings("auto scale\n      CH " ("Variable Name in"), w448) -> (w451:string)
            n151 = Concatenate Strings("Min Max Channel " ("Variable Name in"), w448) -> (w439:string)
            n152 = call "IMAQ Histograph"("Image"=w454) -> ("Histogram Graph"=w459:T14)  [unwired: 7 in, 3 out]
            n153 = call-poly "GFGpolyGet.vi"("Variable Name in"=w439) -> ("output cluster"=w450:T10)  [unwired: 9 in, 1 out]
            n154 = call-poly "GFGpolyGet.vi"("Variable Name in"=w451) -> ("Boolean Value OUT"=w444:bool)  [unwired: 9 in, 1 out]
            n155 = call-poly "GFGpolyGet.vi"("Variable Name in"=w456) -> ("output cluster"=w457:T10)  [unwired: 9 in, 1 out]
            n156 = Unbundle By Name(w457) -> ("WaveformGraphRef"=w458:refnum<vi>)
            n157 = Unbundle By Name(w450) -> ("SlideRef"=w447:refnum<vi>)
            n158 = property class="WFGraph"(reference=w458, "Value"=w459) -> ()  [unwired: 1 in, 2 out]
            n159 = property class="Slide"(reference=w447) -> (reference out=w442:refnum<vi>, "Value"=w446:variant)  [unwired: 1 in, 1 out]
            n160 = Variant To Data(type=cluster{i32, i32} {0, 2048} ("channel1"), Variant=w446) -> (data=w443:cluster{i32, i32})  [unwired: 1 in, 1 out]
            n161 = Select(t=w441, s=w444, f=w443) -> (s? t:f=w440:cluster{i32, i32})
            n162 = case shown="False" w436 {
              tunnel: w440 -> [w462 w465]
              tunnel: [w461 w463] -> w438
              tunnel: [w460 w464] -> w437
              frame True {
                n163 = Unbundle(w462) -> (w461:i32, w460:i32)
              }
              frame False {
                n164 = Unbundle(w465) -> (w464:i32, w463:i32)
              }
            }
            n165 = property class="Slide"(reference=w442, "Value"=w440) -> ()  [unwired: 1 in, 2 out]
          }
        }
        n166 = Bundle(w410, w409, w408) -> (w407:cluster{i16[][], i32, i32})  [unwired: 1 in]
      }
      n167 = for {
        tunnel: w382 -> [w400] mode=indexing
        tunnel: w381 -> [w399]
        tunnel: w379 -> [w398] mode=indexing
        tunnel: w378 -> [w397]
        tunnel: w377 -> [w395]
        n168 = flat-sequence {
          tunnel: w400 -> [w402]
          tunnel: w399 -> [w404]
          tunnel: w395 -> [w403]
          tunnel: w396 -> [w405]
          frame #0 {
            n169 = call "overlay3channels.vi"("active channels"=w403, "RGB Overlay"=w402, "Array"=w404) -> ("RGB Image Out"=w401:T1)  [unwired: 8 in]
            n170 = call "grid_overlay and calculate grid size.vi"("Image In"=w401) -> ()  [unwired: 10 in, 1 out]
          }
          frame #1 {
            n171 = invoke class="ImageControl" method="Refresh Image"(reference=w405) -> ()  [unwired: 2 in, 3 out]
          }
        }
        n172 = To More Specific Class(target class=w397, reference=w398) -> (specific class reference=w396:refnum<vi>)  [unwired: 1 in, 1 out]
      }
    }
    frame Default {
      n173 = for {
        N: 1 -> [_]
        tunnel: w479 -> [w494]
        tunnel: w478 -> [w493]
        tunnel: w477 -> [w492]
        tunnel: w476 -> [w488]
        tunnel: w474 -> [w497]
        shift-right: [w488] -> _
        shift-left: _ -> [w496]
        tunnel: w473 -> [w487]
        tunnel: w472 -> [w486]
        tunnel: w471 -> [w485]
        tunnel: w470 -> [w484]
        tunnel: w469 -> [w483]
        tunnel: w468 -> [w482]
        tunnel: w467 -> [w481]
        tunnel: w466 -> [w480]
        n174 = Not Equal?(x=w496, y=w488) -> (x != y?=w498:bool)
        n175 = case shown="\"all channels\"" w488 {
          tunnel: w494 -> [_ w506 w520 w537 w554 w566]
          tunnel: w493 -> [_ w507 w521 w538 w555 w565]
          tunnel: [_ w503 w517 w534 w551 w562] -> w490
          tunnel: [_ w502 w516 w533 w550 w563] -> w491
          tunnel: w492 -> [_ w501 w515 w531 w548 w564]
          tunnel: [_ w500 w514 w530 w547 w564] -> w489
          tunnel: w482 -> [_ w499 _ _ _ _]
          tunnel: w483 -> [_ _ _ w529 _ _]
          tunnel: w485 -> [_ _ _ _ w546 _]
          tunnel: w481 -> [_ _ w513 _ _ _]
          tunnel: w484 -> [_ _ w512 _ _ _]
          tunnel: w486 -> [_ _ _ w528 _ _]
          tunnel: w487 -> [_ _ _ _ w545 _]
          frame Default {
          }
          frame "Channel 1" {
            w504 = 4 ("index")
            w505 = 1 ("length")
            n176 = case shown="True" w499 {
              tunnel: w501 -> [_ w511]
              tunnel: [_ w509] -> w500
              frame False {
              }
              frame True {
                n177 = Array Subset(array=w511, index (dim 0)=0 ("index"), length (dim 0)=1 ("length")) -> (w509:i16[][][])  [unwired: 4 in]
              }
            }
            n178 = Array Subset(array=w506, index=w504, length=w505) -> (w502:refnum<vi>[])
            n179 = Array Subset(array=w507, index=w504, length=w505) -> (w503:T1[])
          }
          frame "Channel 2" {
            w518 = 5 ("index")
            w519 = 1 ("length")
            n180 = case shown="True" w512 {
              tunnel: w515 -> [_ w525]
              tunnel: [_ w524] -> w514
              tunnel: w513 -> [_ w522]
              frame False {
              }
              frame True {
                n181 = Subtract(x=1 ("index"), y=w522) -> (x-y=w523:i32)
                n182 = Array Subset(array=w525, index (dim 0)=w523, length (dim 0)=1 ("length")) -> (w524:i16[][][])  [unwired: 4 in]
              }
            }
            n183 = Array Subset(array=w521, index=w518, length=w519) -> (w517:T1[])
            n184 = Array Subset(array=w520, index=w518, length=w519) -> (w516:refnum<vi>[])
          }
          frame "Channel 3" {
            w535 = 1 ("index")
            w536 = 6 ("index")
            n185 = case shown="True" w528 {
              tunnel: 2 ("index") -> [_ w543]
              tunnel: w531 -> [_ w542]
              tunnel: [_ w541] -> w530
              tunnel: w529 -> [_ w539]
              frame False {
              }
              frame True {
                n186 = Subtract(x=w543, y=w539) -> (x-y=w540:i32)
                n187 = Array Subset(array=w542, index (dim 0)=w540, length (dim 0)=1 ("length")) -> (w541:i16[][][])  [unwired: 4 in]
              }
            }
            n188 = Array Subset(array=w537, index=w536, length=w535) -> (w533:refnum<vi>[])
            n189 = Array Subset(array=w538, index=w536, length=w535) -> (w534:T1[])
          }
          frame "Channel 4" {
            w552 = 7 ("index")
            w553 = 1 ("index")
            n190 = case shown="True" w545 {
              tunnel: 3 ("index") -> [_ w560]
              tunnel: w548 -> [_ w559]
              tunnel: [_ w558] -> w547
              tunnel: w546 -> [_ w556]
              frame False {
              }
              frame True {
                n191 = Subtract(x=w560, y=w556) -> (x-y=w557:i32)
                n192 = Array Subset(array=w559, index (dim 0)=w557, length (dim 0)=1 ("length")) -> (w558:i16[][][])  [unwired: 4 in]
              }
            }
            n193 = Array Subset(array=w554, index=w552, length=w553) -> (w550:refnum<vi>[])
            n194 = Array Subset(array=w555, index=w552, length=w553) -> (w551:T1[])
          }
          frame "all channels" {
            w568 = 0 ("index")
            w567 = 4 ("length")
            n195 = Array Subset(array=w566, index=w568, length=w567) -> (w563:refnum<vi>[])
            n196 = Array Subset(array=w565, index=w568, length=w567) -> (w562:T1[])
          }
        }
        n197 = for {
          tunnel: w491 -> [w574] mode=indexing
          tunnel: w490 -> [w576] mode=indexing
          tunnel: w489 -> [w581]
          tunnel: w488 -> [w580]
          tunnel: w497 -> [_]
          tunnel: [w573] -> w495
          tunnel: w480 -> [w571]
          i -> [w573]
          n198 = Index Array(array=w581, index (dim 0)=w573) -> (element=w575:i16[][])  [unwired: 2 in]
          n199 = Increment(x=w573) -> (x+1=w579:i32)
          n200 = flat-sequence {
            tunnel: w575 -> [w583]
            tunnel: w576 -> [w584]
            tunnel: [w584] -> w578
            tunnel: [w583] -> w577
            tunnel: w571 -> [w582]
            tunnel: w578 -> [w593]
            tunnel: w577 -> [w595]
            tunnel: w572 -> [w594]
            tunnel: w574 -> [w592]
            frame #0 {
              n201 = Empty Array?(array=w583) -> (empty?=w585:bool)
              n202 = case shown="False" w585 {
                tunnel: w584 -> [w591 _]
                tunnel: w583 -> [w590 _]
                tunnel: w582 -> [w586 _]
                frame False {
                  n203 = call "IMAQ ArrayToImage"("Image Pixels (I16)"=w590, "Image"=w591) -> ("Image Out"=w589:T1)  [unwired: 8 in, 1 out]
                  n204 = call "grid_overlay and calculate grid size.vi"("Image In"=w589) -> ()  [unwired: 10 in, 1 out]
                  n205 = call "GFG_core.vi"("Variable Name in"="CurrentImageType", "Variant in"=w586, "Action"=enum16{"Init", "Set", "Get", "Clear"}."Set") -> ()  [unwired: 10 in, 7 out]
                }
                frame True {
                }
              }
            }
            frame #1 {
              n206 = call "calculate histogram.vi"("channel no."=w594, "Image Ctrl Ref (as generic class)"=w592, "Image Array"=w595, "Image"=w593) -> ()  [unwired: 8 in]
            }
          }
          n207 = case shown="\"all channels\"" w580 {
            tunnel: [1 2 3 4 w600] -> w572
            tunnel: w579 -> [_ _ _ _ w600]
            frame "Channel 1", Default {
            }
            frame "Channel 2" {
            }
            frame "Channel 3" {
            }
            frame "Channel 4" {
            }
            frame "all channels" {
            }
          }
        }
        n208 = case shown="True" w498 {
          tunnel: w491 -> [_ w570]
          tunnel: w490 -> [_ w569]
          tunnel: w495 -> [_ _]
          frame False {
          }
          frame True {
            n209 = call "set initial zoom.vi"("Image Refs In"=w569, "DisplayRefsIn(generic class)"=w570) -> ()  [unwired: 10 in]
          }
        }
      }
    }
  }
